vi "Handle Error.vi"(8 "error in (no error)":errorcluster, 11 "RootModelPublishesDoubleFloat in":refnum<class "RootModelPublishesDoubleFloat.lvclass">) -> (0 "error out":errorcluster, 2 "stop actor?":bool=TRUE, 3 "RootModelPublishesDoubleFloat out":refnum<class "RootModelPublishesDoubleFloat.lvclass">)   [LabVIEW 2017, in "RootModelPublishesDoubleFloat.lvlib" / "RootModelPublishesDoubleFloat.lvclass"]
doc: "(<B>Filename</B>: Actor Framework.lvlib:Actor.lvclass:Handle Error.vi)\n\nDefines how the actor handles an error that occurred while processing a message. By default, this method does nothing except stop the actor."
uses:
  RootModelPublishesDoubleFloat.lvclass
  RootModelPublishesDoubleFloat.lvclass/RootModelPublishesDoubleFloat.ctl
  Source/RootModel/RootModel/RootModel.lvclass
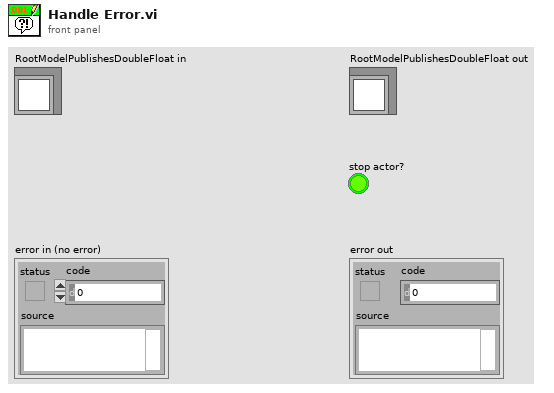
[diagram p1: front panel]
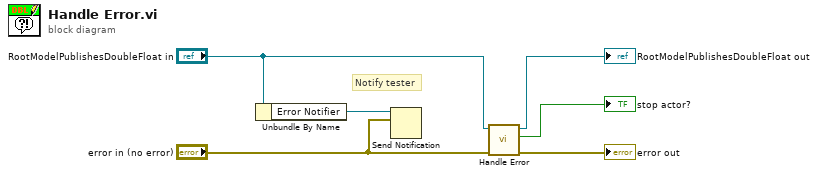
[diagram p0: block diagram]
diagram:
  # "Notify tester"
  n1 = Unbundle By Name("RootModelPublishesDoubleFloat in") -> ("Error Notifier"=w2:refnum<notifier>)
  n2 = Send Notification(notification="error in (no error)", notifier=w2) -> ()  [unwired: 1 in, 2 out]
  n3 = call-parent "Handle Error.vi"("error in (no error)"="error in (no error)", "IModel in"="RootModelPublishesDoubleFloat in") -> ("error out"=→"error out":errorcluster, "stop actor?"=→"stop actor?":bool, "IModel out"=→"RootModelPublishesDoubleFloat out":refnum<class "RootModelPublishesDoubleFloat.lvclass">)  [unwired: 7 in]
